vi "Refresh Display.vi"(8 "error in (no error)":errorcluster, 11 "FunctionGenerator in":refnum<class "FunctionGenerator.lvclass">) -> (0 "error out":errorcluster, 3 "FunctionGenerator out":refnum<class "FunctionGenerator.lvclass">)   [LabVIEW 2019, in "FunctionGenerator.lvlib" / "FunctionGenerator.lvclass"]
uses:
  Library/FunctionGenerator.lvclass
  Library/FunctionGenerator.lvclass/FunctionGenerator.ctl
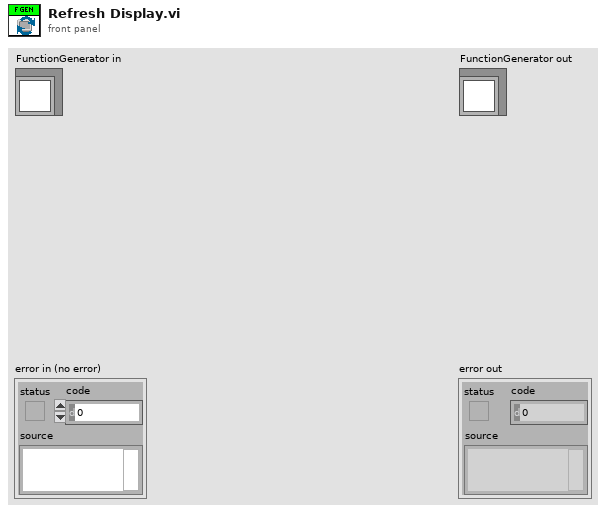
[diagram p1: front panel]
types:
  T1 = typedef "FunctionGenerator.lvlib/FunctionGenerator.lvclass/WaveformSettings.ctl" = cluster{"Frequency":dbl, "Amplitude":dbl, "Offset":dbl, "Phase":dbl, "Symmetry":dbl, "Pulse Width":dbl, "Rise Time":dbl, "Fall Time":dbl, "Mode":T2, "Termination":enum16{"50_Ohm", "High_Z"}, "Output":bool}
  T2 = typedef "FunctionGenerator.lvlib/FunctionGenerator.lvclass/WaveformMode.ctl" = enum16{"Sine", "Square", "Ramp", "Pulse", "Arbitrary", "Triangle", "Noise", "DC"}
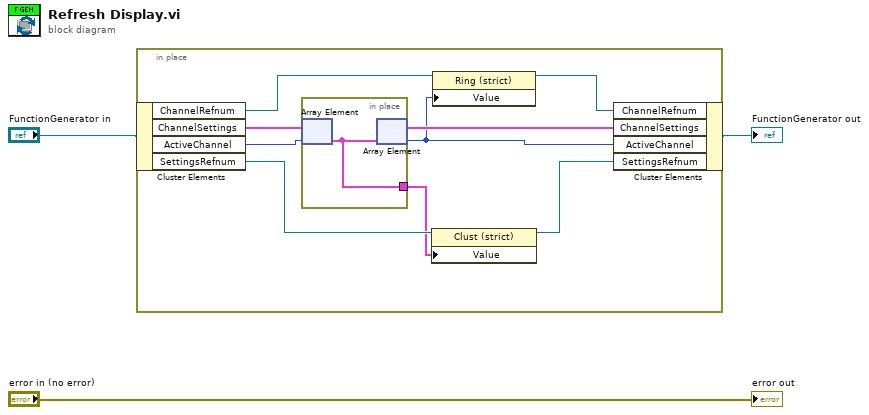
[diagram p0: block diagram]
diagram:
  n1 = in-place {
    n2 = in-place-cluster #1("FunctionGenerator in") -> ("ChannelRefnum"=w9:refnum<vi>, "ChannelSettings"=w12:T1[], "ActiveChannel"=w11:i32, "SettingsRefnum"=w6:refnum<vi>)
    n3 = in-place {
      in-place-border: [w13] -> w4
      n4 = in-place-array #2(w12, w11) -> (w13:T1)
      n5 = in-place-array #2(w13) -> (w10:T1[], w8:i32)
    }
    n6 = property class="Clust (strict)"(reference=w6, "Value"=w4) -> (reference out=w5:refnum<vi>)  [unwired: 1 in, 1 out]
    n7 = property class="Ring (strict)"(reference=w9, "Value"=w8) -> (reference out=w7:refnum<vi>)  [unwired: 1 in, 1 out]
    n8 = in-place-cluster #1("ChannelRefnum"=w7, "ChannelSettings"=w10, "ActiveChannel"=w8, "SettingsRefnum"=w5) -> (→"FunctionGenerator out":refnum<class "FunctionGenerator.lvclass">)
  }
  "error out" <- "error in (no error)"
